vi "test_Format Numeric To String_double to string using native endian.vi"(8 "error in (no error)":errorcluster, 11 "TestCase in":refnum<class "Instrument Addon Unit Tests.lvclass">) -> (0 "error out":errorcluster, 3 "TestCase out":refnum<class "Instrument Addon Unit Tests.lvclass">)   [LabVIEW 2020, in "Instrument Addon Unit Tests.lvclass"]
uses:
  Instrument Addon Unit Tests.lvclass
  Addon/Addon Shared/Types/Endian.ctl
  <vilib>/addons/_JKI Toolkits/VI Tester/TestCase.llb/TestCase.lvclass
  Addon/Addon Shared/Instrument Addon Shared.lvlib
  C:/Program Files (x86)/National Instruments/LabVIEW 2020/vi.lib/addons/_JKI Toolkits/VI Tester/TestCase.llb/TestCase.lvclass
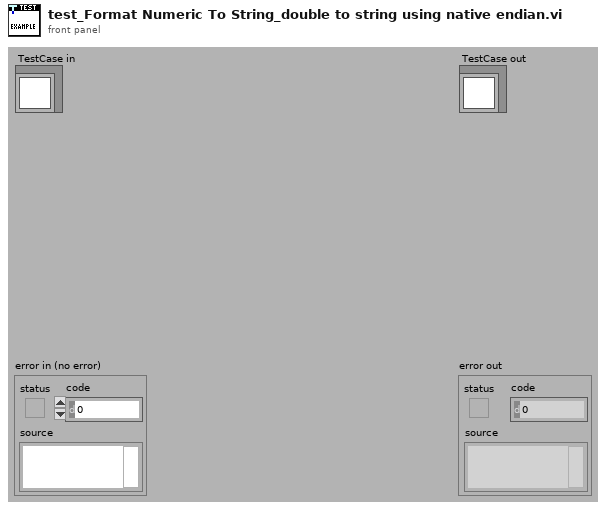
[diagram p1: front panel]
types:
  T1 = typedef "Instrument Addon Shared.lvlib/Endian.ctl" = enum16{"Native", "Little", "Big"}
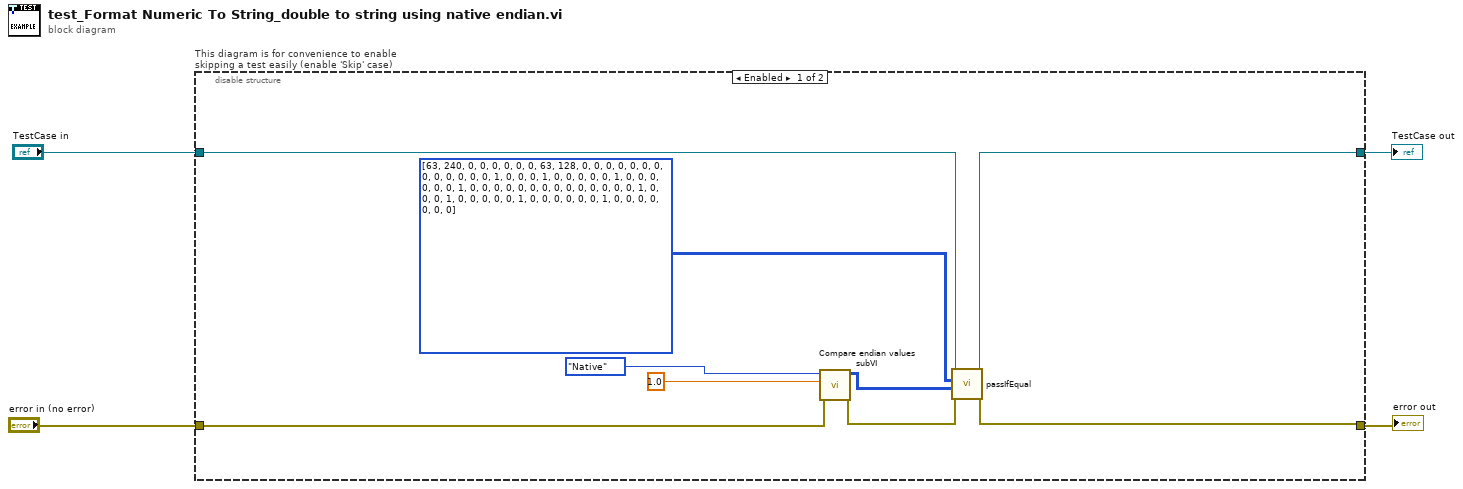
[diagram p0: block diagram]
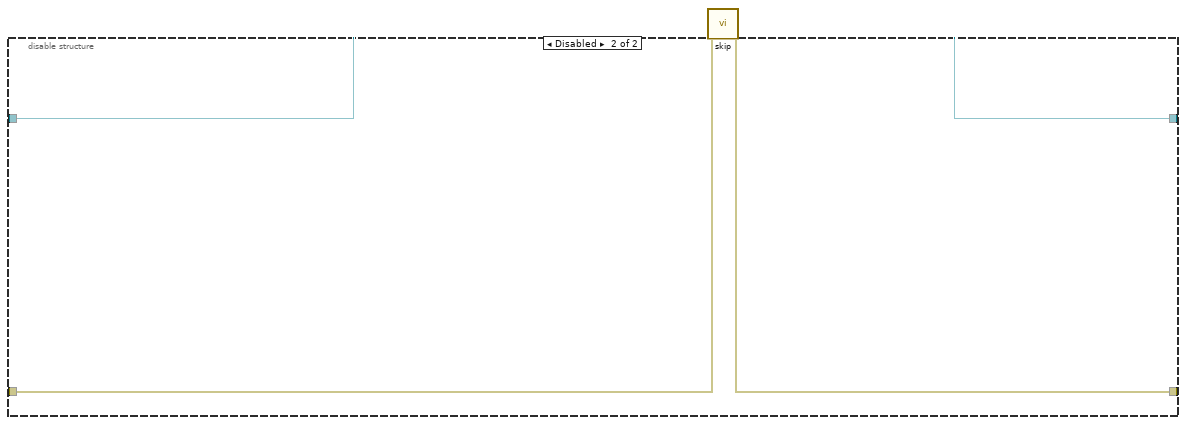
[diagram p2: hidden frame]
diagram:
  n1 = disable-structure "This diagram is for convenience to enable skipping a test easily (enable 'Skip' case)" shown="Enabled" {
    disable-tunnel: "TestCase in" -> [w13 w17]
    disable-tunnel: [w12 w15] -> w1
    disable-tunnel: [w11 w16] -> w3
    disable-tunnel: "error in (no error)" -> [w8 w14]
    frame Enabled {
      n2 = call "Compare endian values subVI.vi"("error in (no error)"=w8, "Numeric"=1.0, "Endian"=Endian."Native") -> ("error out"=w7:errorcluster, "Values Out"=w6:u8[][])  [unwired: 7 in]
      n3 = call-dynamic "passIfEqual.vi"("error in (no error)"=w7, "y"=w6, "x"=u8[][] [[63, 240, 0, 0, 0, 0, 0, 0], [63, 128, 0, 0, 0, 0, 0, 0], [0, 0, 0, 0, 0, 0, 0, 1], [0, 0, 0, 1, 0, 0, 0, 0], [0, 1, 0, 0, 0, 0, 0, 0], [1, 0, 0, 0, 0, 0, 0, 0], [0, 0, 0, 0, 0, 0, 0, 1], [0, 0, 0, 1, 0, 0, 0, 0], [0, 1, 0, 0, 0, 0, 0, 0], [1, 0, 0, 0, 0, 0, 0, 0]] ("unsigned byte array"), "TestCase in"=w13) -> ("error out"=w11:errorcluster, "TestCase out"=w12:refnum<class "Instrument Addon Unit Tests.lvclass">)  [unwired: 6 in]
    }
    frame Disabled {
      # "skip test result while test is under development"
      n4 = call <vilib>:"skip.vi"("error in (no error)"=w14, "TestCase in"=w17) -> ("error out"=w16:errorcluster, "TestCase out"=w15:refnum<class "Instrument Addon Unit Tests.lvclass">)  [unwired: 8 in]
    }
  }
  "error out" <- w3
  "TestCase out" <- w1
